vi "_FPGA Read Data.vi"(4 "error in":errorcluster, 5 "Read Mode (Do Read)":T1=enum."Do Read", 6 "Address":u16) -> (0 "error out":errorcluster, 2 "Data":u32)   [LabVIEW 2015]
uses:
  Type/_RW Status.ctl
  Type/_FPGA Indicator.ctl
  _RT Global.vi
  <vilib>/Utility/error.llb/Error Cluster From Error Code.vi
  <vilib>/rvi/errors/niLvFpgaAdjustHostInterfaceError.vi
  <vilib>/rvi/interface/nirviReadWriteControl/nirviReadWriteControl.xnode
  Type/FPGA Typedef.ctl
  FPGA Bitfiles/FPGA9607.lvbitx
  NiFpgaLv.dll
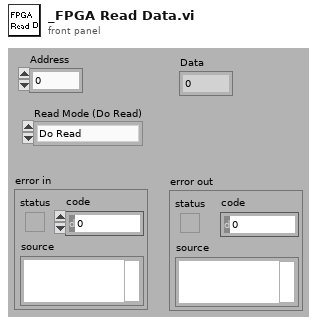
[diagram p1: front panel]
types:
  T1 = typedef "_RW Status.ctl" = enum8{"Done", "Do Read", "Do Write", "Set Latch1", "Set Latch2", "Set Latch3", "Set Latch4", "RP ON", "EL ON", "Serial Send", "Set LC Out", "Get LC In", "Read VAC", "Table Test", "Get Interlock", "Do Read2", "Do Write2"}
  T2 = typedef "Semaphore RefNum" = refnum<k1>
  T3 = typedef "_FPGA Indicator.ctl" = enum16{"Done", "Ready", "Count Available", "SendSerial", "LED State"}
  T4 = typedef "FPGA Typedef.ctl" = refnum<k20>
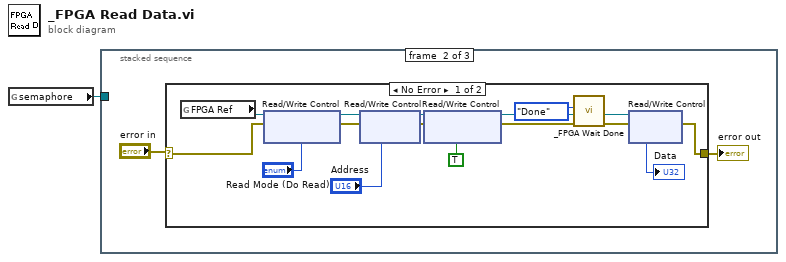
[diagram p0: block diagram]
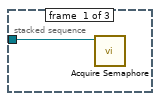
[diagram p2: hidden frame]
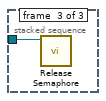
[diagram p4: hidden frame]
diagram:
  n1 = global read "_RT Global.vi" "semaphore"() -> (w1:T2)
  n2 = stacked-sequence {
    tunnel: w1 -> [w2 _ w21]
    frame #0 {
      n3 = call <vilib>:"Acquire Semaphore.vi"("semaphore"=w2) -> ()  [unwired: 2 in, 5 out]
    }
    frame #1 {
      n4 = case shown="No Error" "error in" {
        selector: "error in" -> [w13 w20]
        tunnel: [w8 w20] -> w3
        frame No Error {
          n5 = global read "_RT Global.vi" "FPGA Ref"() -> (w6:T4)
          n6 = xnode "Read/Write Control"("FPGA VI Reference In"=w6, "error in"=w13, "R/W Status"="Read Mode (Do Read)") -> ("FPGA VI Reference Out"=w15:T4, "error out"=w16:errorcluster)
          n7 = xnode "Read/Write Control"("FPGA VI Reference In"=w15, "error in"=w16, "Address"="Address") -> ("FPGA VI Reference Out"=w12:T4, "error out"=w11:errorcluster)
          n8 = xnode "Read/Write Control"("FPGA VI Reference In"=w12, "error in"=w11, "Read/Write"=TRUE ("Data Written")) -> ("FPGA VI Reference Out"=w5:T4, "error out"=w9:errorcluster)
          n9 = call "_FPGA Wait Done.vi"("error in"=w9, "Indicator"=_FPGA_Indicator."Done") -> ("error out"=w7:errorcluster)  [unwired: 3 in, 2 out]
          n10 = xnode "Read/Write Control"("FPGA VI Reference In"=w5, "error in"=w7) -> ("error out"=w8:errorcluster, "Data"=→"Data":u32)  [unwired: 1 out]
        }
        frame Error {
        }
      }
      "error out" <- w3
    }
    frame #2 {
      n11 = call <vilib>:"Release Semaphore.vi"("semaphore"=w21) -> ()  [unwired: 1 in, 6 out]
    }
  }
